vi "Replace_NaNs.vi"(10 "Array":dbl[](array[numeric]), 11 "Replacement":dbl) -> (3 "Array Out":dbl[](array[numeric]))   [LabVIEW 2022 SP3]
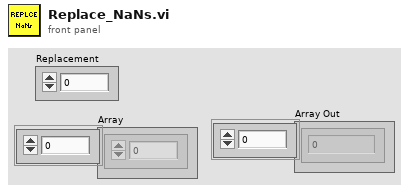
[diagram p1: front panel]
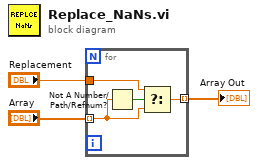
[diagram p0: block diagram]
diagram:
  n1 = for {
    tunnel: "Array" -> [w6] mode=indexing
    tunnel: [w5] -> w2 mode=indexing
    tunnel: "Replacement" -> [w4]
    n2 = Not A Number/Path/Refnum?(number/path/refnum=w6) -> (NaN/Path/Refnum?=w7:bool)
    n3 = Select(t=w4, s=w7, f=w6) -> (s? t:f=w5:dbl)
  }
  "Array Out" <- w2
